vi "FindConnection.vi"(8 "Connection number":i32, 10 "Connections":T1[](array[typedef])) -> (0 "Found?":bool, 1 "Connection Window's Enqueuer":refnum<class "Message Enqueuer.lvclass">, 2 "Connection Handlers's Enqueuer":refnum<class "Message Enqueuer.lvclass">, 3 "Connection index":i32)   [LabVIEW 2023, in "TCP_Server.lvlib" / "TCP_Server.lvclass"]
uses:
  TCP_Server.lvclass
  TypeDeclarations/ServerConnection.ctl
  <vilib>/ActorFramework/Message Enqueuer/Message Enqueuer.lvclass
  TCP_Server.lvclass/TCP_Server.ctl
  TCP_Server.lvlib
  TCP_Listener/TypeDefinitions/ConnectionInformation.ctl
  TCP_Listener/TCP_Listener.lvlib
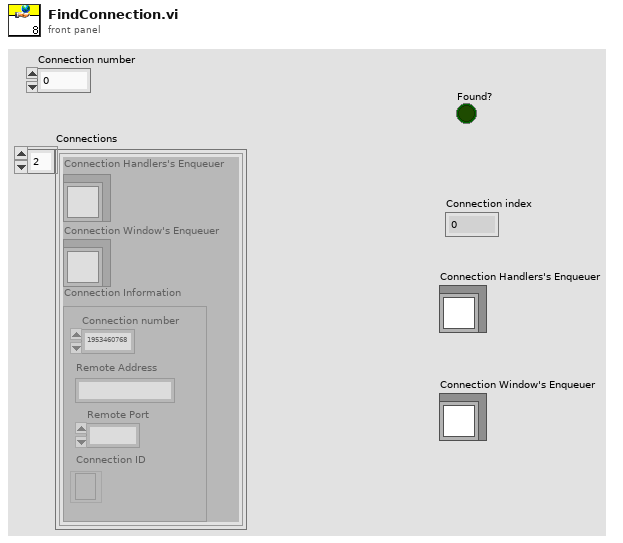
[diagram p1: front panel]
types:
  T1 = typedef "TCP_Server.lvlib/ServerConnection.ctl" = cluster{"Connection Handlers's Enqueuer":refnum<class "Message Enqueuer.lvclass">, "Connection Window's Enqueuer":refnum<class "Message Enqueuer.lvclass">, "Connection Information":T2}
  T2 = typedef "TCP_Listener.lvlib/ConnectionInformation.ctl" = cluster{"Connection number":i32, "Remote Address":string, "Remote Port":u16, "Connection ID":refnum<k5>}
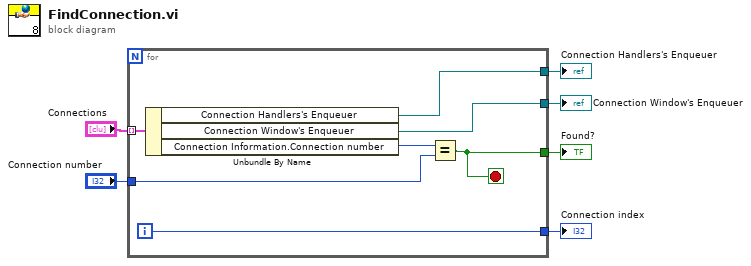
[diagram p0: block diagram]
diagram:
  n1 = for {
    tunnel: "Connections" -> [w13] mode=indexing
    tunnel: "Connection number" -> [w11]
    tunnel: [w10] -> w4
    tunnel: [w9] -> w3
    tunnel: [w8] -> w2
    tunnel: [w7] -> w1
    i -> [w9]
    stop <- w10 stop-if-true
    n2 = Unbundle By Name(w13) -> ("Connection Handlers's Enqueuer"=w8:refnum<class "Message Enqueuer.lvclass">, "Connection Window's Enqueuer"=w7:refnum<class "Message Enqueuer.lvclass">, "Connection Information.Connection number"=w12:i32)
    n3 = Equal?(x=w12, y=w11) -> (x = y?=w10:bool)
  }
  "Connection index" <- w3
  "Found?" <- w4
  "Connection Handlers's Enqueuer" <- w2
  "Connection Window's Enqueuer" <- w1
